vi "Display All Idle.vi"(8 "error in (no error)":errorcluster, 11 "Application in":refnum<class "Application.lvclass">) -> (0 "error out":errorcluster, 3 "Application out":refnum<class "Application.lvclass">)   [LabVIEW 2017, in "Application.lvlib" / "Application.lvclass"]
doc: "Updates all UUTs in the Running state to display the status as \"Idle\". Handy for iterating through a serial test and showing all units Idle except the one performing the test."
uses:
  Application.lvclass
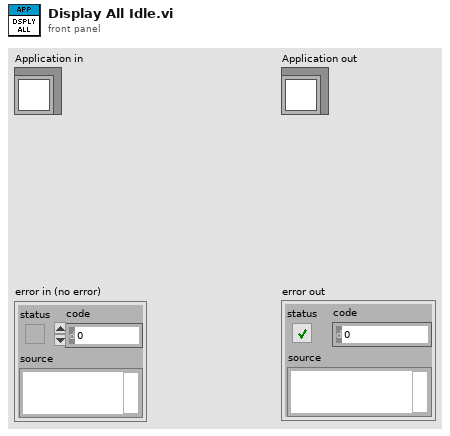
[diagram p1: front panel]
types:
  T1 = cluster{"Serial Number Reference":refnum<vi>, "Status Message Reference":refnum<vi>, "Position":u32}[]
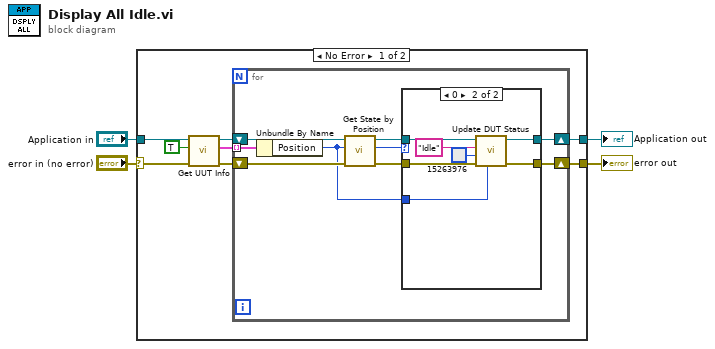
[diagram p0: block diagram]
diagram:
  n1 = case shown="No Error" "error in (no error)" {
    selector: "error in (no error)" -> [w9 w31]
    tunnel: [w12 w32] -> w4
    tunnel: "Application in" -> [w10 w32]
    tunnel: [w11 w31] -> w1
    frame No Error {
      n2 = call-dynamic "Get UUT Info.vi"("error in (no error)"=w9, "Scanned Only (false)"=TRUE, "Application in"=w10) -> ("error out"=w7:errorcluster, "All UUTs"=w6:T1, "Application out"=w8:refnum<class "Application.lvclass">)  [unwired: 6 in]
      n3 = for {
        shift-right: [w21] -> w12
        shift-left: w8 -> [w19]
        tunnel: w6 -> [w20] mode=indexing
        shift-right: [w15] -> w11
        shift-left: w7 -> [w16]
        n4 = Unbundle By Name(w20) -> ("Position"=w13:u32)
        n5 = call-dynamic "Get State by Position.vi"("error in (no error)"=w16, "Position"=w13, "Application in"=w19) -> ("error out"=w14:errorcluster, "State"=w17:u32, "Application out"=w18:refnum<class "Application.lvclass">)  [unwired: 6 in]
        n6 = case shown="0" w17 {
          tunnel: [w23 w30] -> w21
          tunnel: w18 -> [w23 w29]
          tunnel: [w22 w27] -> w15
          tunnel: w14 -> [w22 w28]
          tunnel: w13 -> [_ w24]
          frame Default {
          }
          frame 0 {
            n7 = call "Update DUT Status.vi"("Position"=w24, "error in (no error)"=w28, "BG Color"=u32 15263976, "Message ('')"="Idle", "Application in"=w29) -> ("error out"=w27:errorcluster, "Application out"=w30:refnum<class "Application.lvclass">)  [unwired: 5 in]
          }
        }
      }
    }
    frame Error {
    }
  }
  "Application out" <- w4
  "error out" <- w1
